vi "JustTest.vi"() -> ()   [LabVIEW 2020]
panel:
  out "array":string[](array[string])
  # "PPDU_Power_Mean : 54"
  # "EVM_ALL_Carrier_Mean:25"
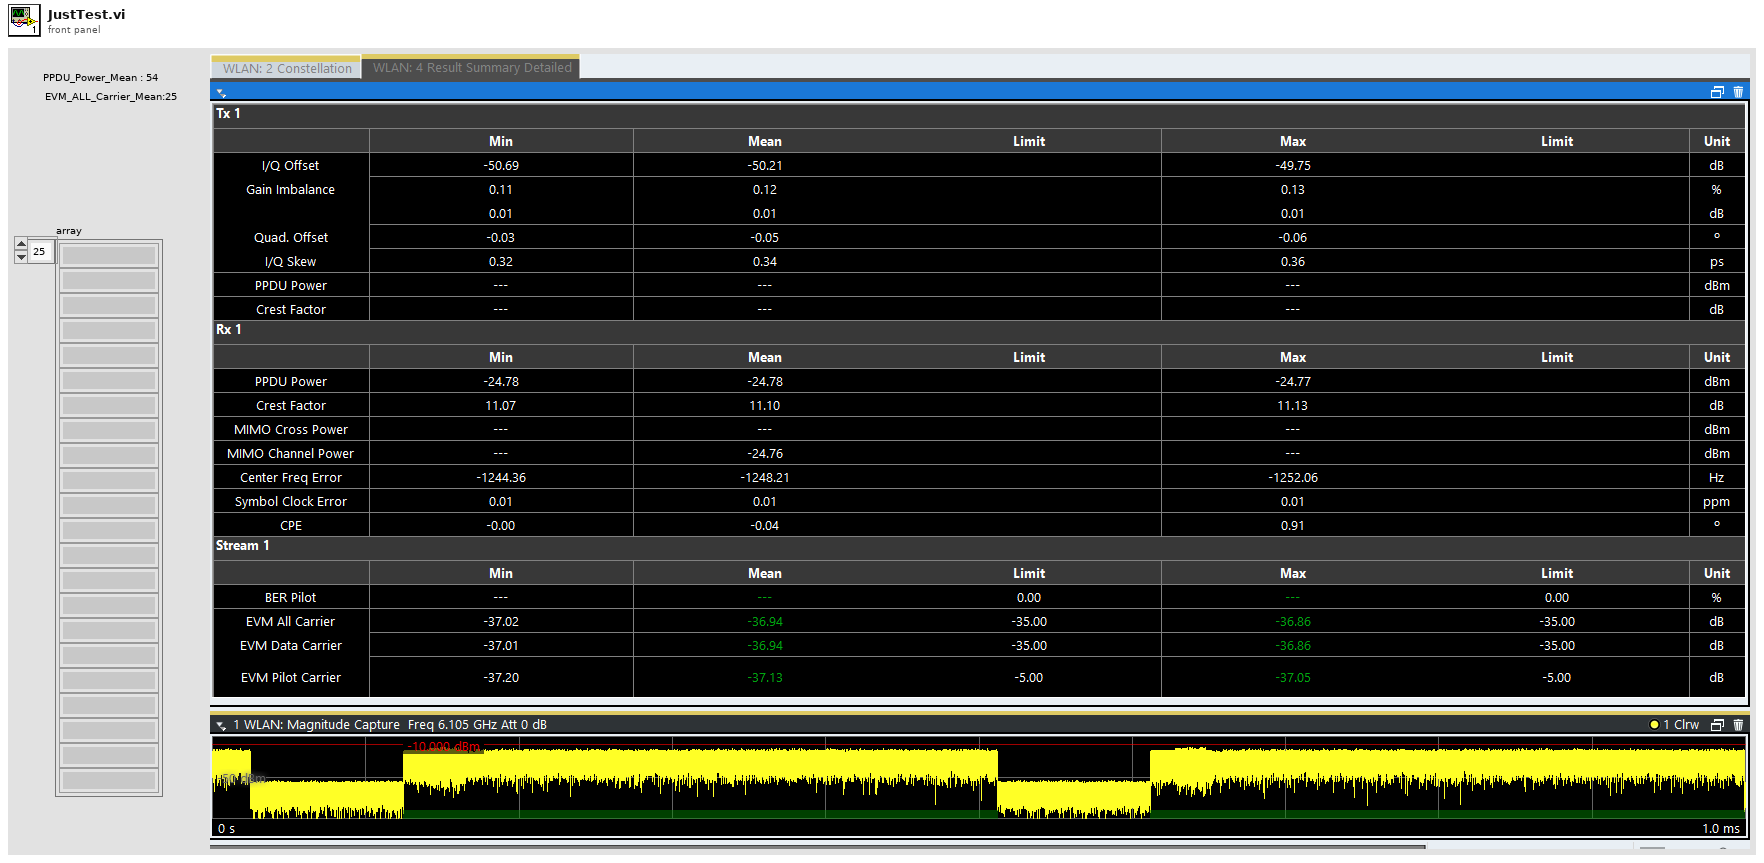
[diagram p1: front panel]
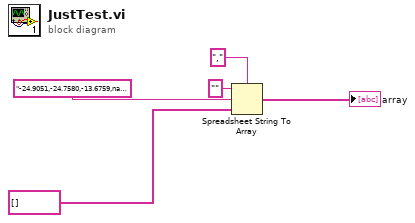
[diagram p0: block diagram]
diagram:
  n1 = Spreadsheet String To Array(delimiter (Tab)=",", format string="", spreadsheet string="-24.9051,-24.7580,-13.6759,nan,nan,nan,nan,nan,nan,-1244.3610,-1248.2117,-1252.0623,0.0121,0.0134,0.0147,nan,nan,nan,nan,nan,nan,nan,nan,nan,-37.0159,-36.9393,-36.8634,-37.0129,-36.9363,-36.8605,-37.2036,-37.1254,-37.0479,nan,nan,nan,nan,nan,nan,nan,nan,nan,nan,nan,nan,nan,nan,nan,nan,nan,nan,nan,nan,-24.7766,-24.7757,-24.7748,11.0674,11.0997,11.1319,-1244.3610,-1248.2117,-1252.0623,0.0121,0.0134,0.0147,-50.6879,-50.2052,-49.7479,0.0098,0.0104,0.0109,-0.0324,-0.0481,-0.0638,-37.0159,-36.9393,-36.8634,-37.0129,-36.9363,-36.8605,-37.2036,-37.1254,-37.0479,nan,nan,nan,0.3233,0.3427,0.3620,nan,nan,nan,-0.0016,-0.0354,0.9123,nan,-24.7613,nannan,nan", array type (2D Dbl)=string[] []) -> (array=→"array":string[])
